vi "AlgorithmLeftGoal - Copy.vi"(0 "MatchBallX":dbl, 1 "MatchBallY":dbl, 2 "D1 X COM":dbl, 3 "D1Y COM":dbl, 4 "D2 X COM":dbl, 5 "D2 Y COM":dbl) -> (9 "RW":cluster{"kRW":dbl, "CoRW":dbl, "type":dbl}, 11 "LW":cluster{"kLW":dbl, "CoLW":dbl, "type":dbl}, 13 "output cluster":T1, 14 "Theta LG,LW":dbl, 15 "aRW":dbl, 16 "aS":dbl, 17 "min x":dbl, 18 "min x2":dbl, 19 "min x3":dbl)   [LabVIEW 2014]
panel:
  out "xD2BotS":dbl
  out "xD2ComS":dbl
  out "xD1BotS":dbl
  out "xD1ComS":dbl
  out "xD2BotR":dbl
  out "xD2ComR":dbl
  out "xD1BotR":dbl
  out "xD1ComR":dbl
  out "D2 X Bot fit 2":dbl
  out "D2 X Com fit":dbl
  out "D1 X Bot fit":dbl
  out "D1 X Com fit":dbl
  # "LOGIC"
  # "Left Goal"
  # "STRAIGHT"
  # "Left wall"
  # "Right Wall"
  # "Straight"
  # "sending data"
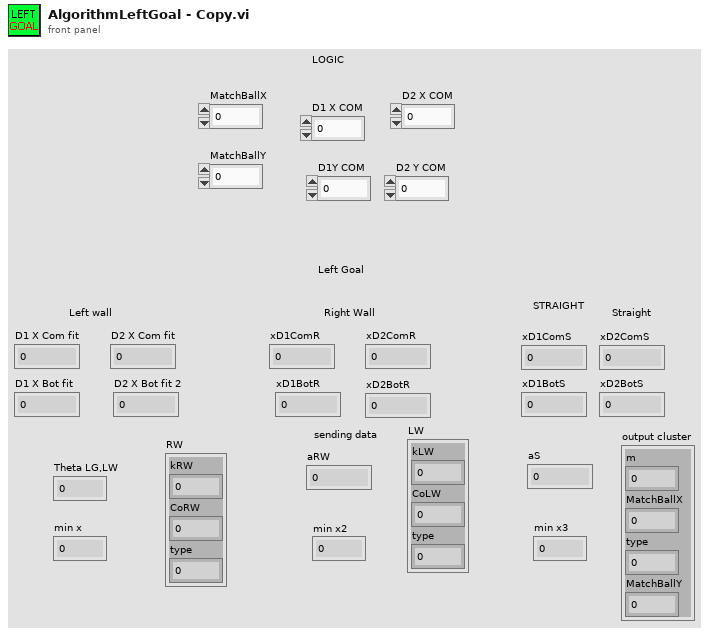
[diagram p1: front panel]
types:
  T1 = cluster{"m":dbl, "MatchBallX":dbl, "type":dbl, "MatchBallY":dbl}
  T2 = cluster{"m":dbl, "MatchBallX":dbl, "y":dbl, "MatchBallY":dbl}
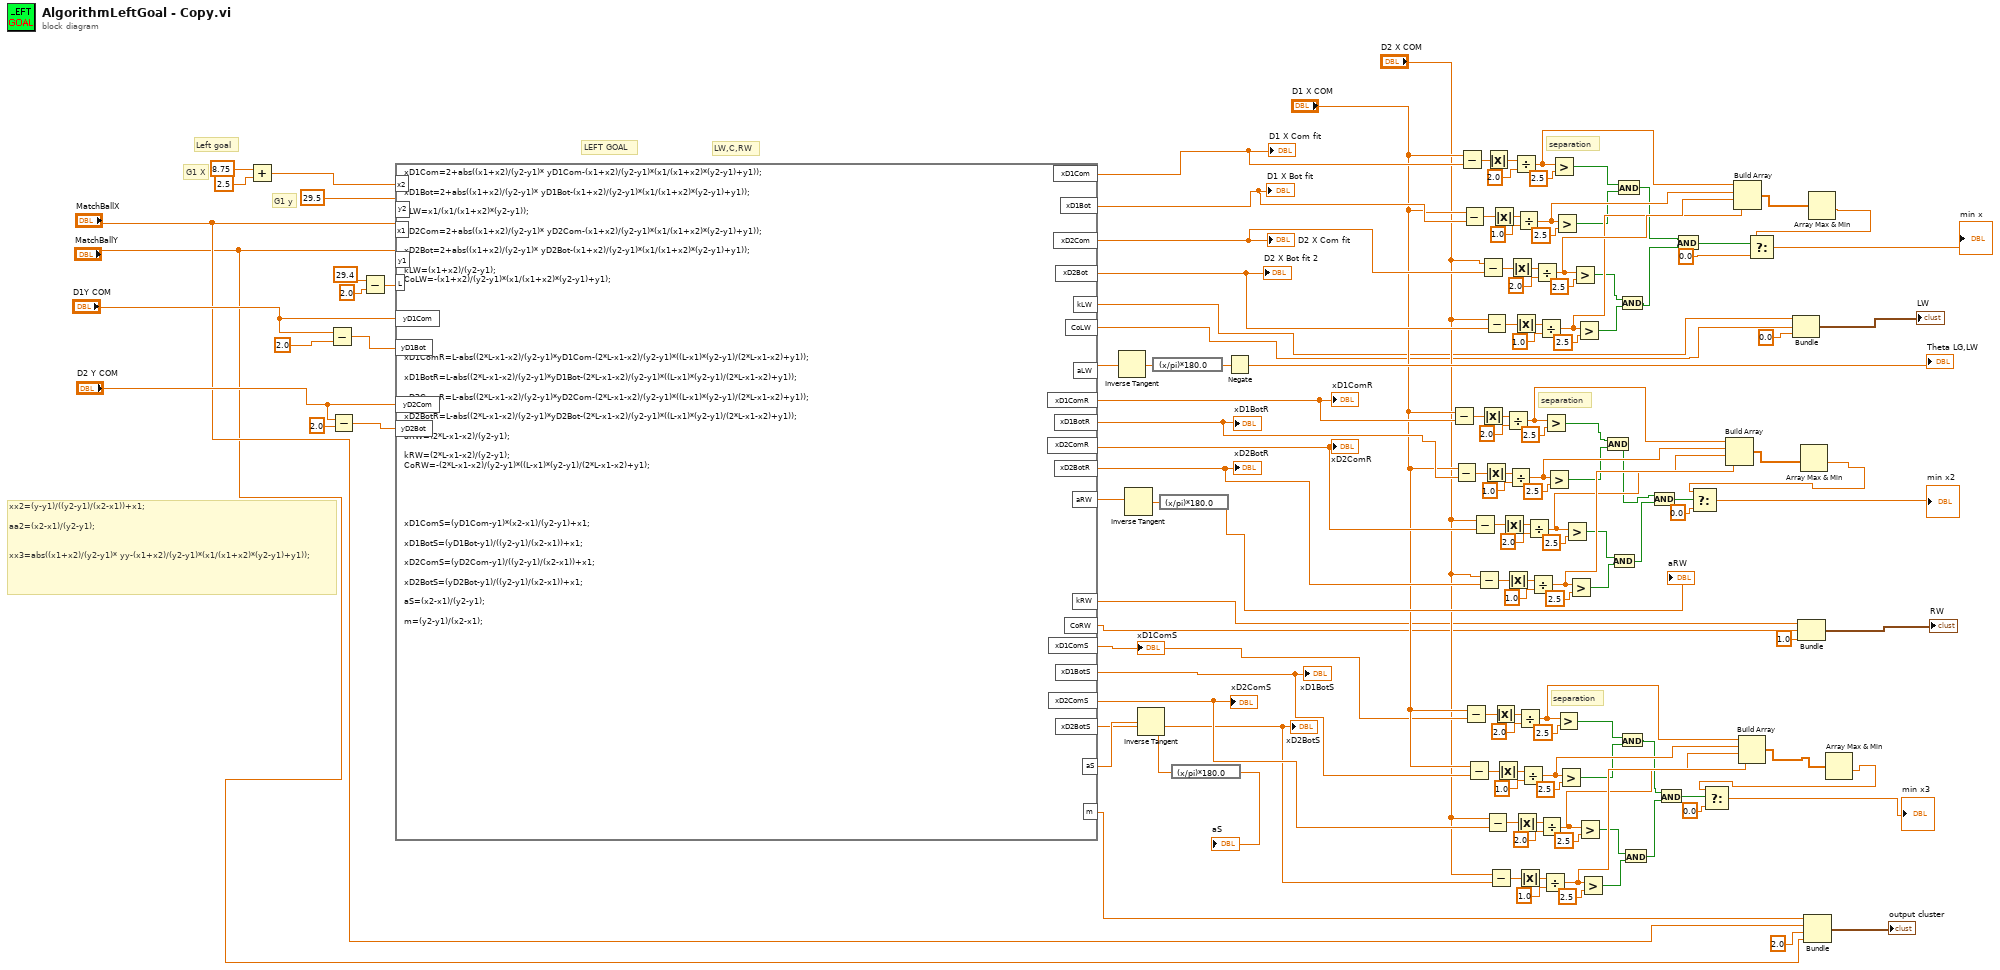
[diagram p0: block diagram]
diagram:
  # "LW,C,RW"
  # "separation"
  # "separation"
  # "separation"
  # "LEFT GOAL"
  # "xx2=(y-y1)/((y2-y1)/(x2-x1))+x1;\n\naa2=(x2-x1)/(y2-y1);\n\n\nxx3=abs((x1+x2)/(y2-y1)* yy-(x1+x2)/(y2-y1)*(x1/(x1+x2)*(y2-y1)+y1));"
  # "Left goal"
  # "G1 y"
  # "G1 X"
  n1 = Add(x=8.75, y=2.5) -> (x+y=w140:dbl)
  n2 = Subtract(x="D1Y COM", y=2.0) -> (x-y=w135:dbl)
  n3 = Subtract(x="D2 Y COM", y=2.0) -> (x-y=w130:dbl)
  n4 = Subtract(x=29.4 ("input variable"), y=2.0) -> (x-y=w15:dbl)
  n5 = formula code="xD1Com=2+abs((x1+x2)/(y2-y1)* yD1Com-(x1+x2)/(y2-y1)*(x1/(x1+x2)*(y2-y1)+y1));\n\nxD1Bot=2+abs((x1+x2)/(y2-y1)* yD1Bot-(x1+x2)/(y2-y1)*(x1/(x1+x2)*(y2-y1)+y1));\n\naLW=x1/(x1/(x1+x2)*(y2-y1));\n\nxD2Com=2+abs((x1+x2)/(y2-y1)* yD2Com-(x1+x2)/(y2-y1)*(x1/(x1+x2)*(y2-y1)+y1));\n\nxD2Bot=2+abs((x1+x2)/(y2-y1)* yD2Bot-(x1+x2)/(y2-y1)*(x1/(x1+x2)*(y2-y1)+y1));\n\nkLW=(x1+x2)/(y2-y1);\nCoLW=-(x1+x2)/(y2-y1)*(x1/(x1+x2)*(y2-y1)+y1);\n\n\n\n\n\n\n\nxD1ComR=L-abs((2*L-x1-x2)/(y2-y1)*yD1Com-(2*L-x1-x2)/(y2-y1)*((L-x1)*(y2-y1)/(2*L-x1-x2)+y1));\n\nxD1BotR=L-abs((2*L-x1-x2)/(y2-y1)*yD1Bot-(2*L-x1-x2)/(y2-y1)*((L-x1)*(y2-y1)/(2*L-x1-x2)+y1));\n\nxD2ComR=L-abs((2*L-x1-x2)/(y2-y1)*yD2Com-(2*L-x1-x2)/(y2-y1)*((L-x1)*(y2-y1)/(2*L-x1-x2)+y1));\n\nxD2BotR=L-abs((2*L-x1-x2)/(y2-y1)*yD2Bot-(2*L-x1-x2)/(y2-y1)*((L-x1)*(y2-y1)/(2*L-x1-x2)+y1));\n\naRW=(2*L-x1-x2)/(y2-y1);\n\nkRW=(2*L-x1-x2)/(y2-y1);\nCoRW=-(2*L-x1-x2)/(y2-y1)*((L-x1)*(y2-y1)/(2*L-x1-x2)+y1);\n\n\n\n\n\nxD1ComS=(yD1Com-y1)*(x2-x1)/(y2-y1)+x1;\n\nxD1BotS=(yD1Bot-y1)/((y2-y1)/(x2-x1))+x1;\n\nxD2ComS=(yD2Com-y1)/((y2-y1)/(x2-x1))+x1;\n\nxD2BotS=(yD2Bot-y1)/((y2-y1)/(x2-x1))+x1;\n\naS=(x2-x1)/(y2-y1);\n\nm=(y2-y1)/(x2-x1);"("x1"="MatchBallX", "x2"=w140, "y2"=29.5, "y1"="MatchBallY", "yD1Com"="D1Y COM", "yD2Com"="D2 Y COM", "yD1Bot"=w135, "yD2Bot"=w130, "L"=w15) -> ("xD1Com"=w123:dbl, "aLW"=w138:dbl, "xD1Bot"=w109:dbl, "xD2Com"=w114:dbl, "xD2Bot"=w104:dbl, "xD1ComR"=w77:dbl, "xD1BotR"=w76:dbl, "xD2ComR"=w75:dbl, "xD2BotR"=w74:dbl, "aRW"=w128:dbl, "xD1ComS"=w51:dbl, "aS"=w124:dbl, "xD1BotS"=w50:dbl, "xD2BotS"=w48:dbl, "xD2ComS"=w49:dbl, "kLW"=w13:dbl, "CoLW"=w12:dbl, "kRW"=w9:dbl, "CoRW"=w8:dbl, "m"=w5:dbl)
  "D1 X Com fit" <- w123
  "D1 X Bot fit" <- w109
  "D2 X Com fit" <- w114
  "D2 X Bot fit 2" <- w104
  "xD1ComR" <- w77
  "xD1BotR" <- w76
  "xD2ComR" <- w75
  "xD2BotR" <- w74
  "xD1ComS" <- w51
  "xD1BotS" <- w50
  "xD2ComS" <- w49
  "xD2BotS" <- w48
  n6 = Inverse Tangent(1:w138) -> (0:w139:dbl)
  n7 = Inverse Tangent(1:w128) -> (0:w129:dbl)
  n8 = Inverse Tangent(1:w124) -> (0:w125:dbl)
  n9 = expression code="(x/pi)*180.0" ("radians to degrees")(w139) -> (w136:dbl)
  n10 = expression code="(x/pi)*180.0" ("radians to degrees")(w129) -> (→"aRW":dbl)
  n11 = expression code="(x/pi)*180.0" ("radians to degrees")(w125) -> (→"aS":dbl)
  n12 = Negate(x=w136) -> (-x=→"Theta LG,LW":dbl)
  n13 = Subtract(x="D1 X COM", y=w77) -> (x-y=w78:dbl)
  n14 = Subtract(x="D1 X COM", y=w76) -> (x-y=w89:dbl)
  n15 = Subtract(x="D1 X COM", y=w123) -> (x-y=w122:dbl)
  n16 = Subtract(x="D1 X COM", y=w109) -> (x-y=w110:dbl)
  n17 = Subtract(x="D1 X COM", y=w51) -> (x-y=w53:dbl)
  n18 = Subtract(x="D1 X COM", y=w50) -> (x-y=w64:dbl)
  n19 = Subtract(x="D2 X COM", y=w75) -> (x-y=w85:dbl)
  n20 = Subtract(x="D2 X COM", y=w74) -> (x-y=w90:dbl)
  n21 = Subtract(x="D2 X COM", y=w114) -> (x-y=w115:dbl)
  n22 = Absolute Value(x=w78) -> (abs(x)=w79:dbl)
  n23 = Absolute Value(x=w89) -> (abs(x)=w88:dbl)
  n24 = Subtract(x="D2 X COM", y=w104) -> (x-y=w108:dbl)
  n25 = Subtract(x="D2 X COM", y=w49) -> (x-y=w60:dbl)
  n26 = Absolute Value(x=w122) -> (abs(x)=w121:dbl)
  n27 = Subtract(x="D2 X COM", y=w48) -> (x-y=w65:dbl)
  n28 = Absolute Value(x=w110) -> (abs(x)=w111:dbl)
  n29 = Absolute Value(x=w53) -> (abs(x)=w54:dbl)
  n30 = Absolute Value(x=w64) -> (abs(x)=w63:dbl)
  n31 = Absolute Value(x=w85) -> (abs(x)=w84:dbl)
  n32 = Divide(x=w79, y=2.0) -> (x/y=w95:dbl)
  n33 = Absolute Value(x=w90) -> (abs(x)=w91:dbl)
  n34 = Divide(x=w88, y=1.0) -> (x/y=w96:dbl)
  n35 = Absolute Value(x=w115) -> (abs(x)=w116:dbl)
  n36 = Divide(x=w121, y=2.0) -> (x/y=w102:dbl)
  n37 = Absolute Value(x=w108) -> (abs(x)=w107:dbl)
  n38 = Absolute Value(x=w60) -> (abs(x)=w59:dbl)
  n39 = Divide(x=w111, y=1.0) -> (x/y=w101:dbl)
  n40 = Divide(x=w54, y=2.0) -> (x/y=w70:dbl)
  n41 = Absolute Value(x=w65) -> (abs(x)=w66:dbl)
  n42 = Divide(x=w63, y=1.0) -> (x/y=w71:dbl)
  n43 = Divide(x=w84, y=2.0) -> (x/y=w97:dbl)
  n44 = Divide(x=w91, y=1.0) -> (x/y=w98:dbl)
  n45 = Divide(x=w116, y=2.0) -> (x/y=w100:dbl)
  n46 = Divide(x=w107, y=1.0) -> (x/y=w99:dbl)
  n47 = Divide(x=w59, y=2.0) -> (x/y=w72:dbl)
  n48 = Divide(x=w66, y=1.0) -> (x/y=w73:dbl)
  n49 = Greater?(x=w95, y=2.5) -> (0:w34:bool)
  n50 = Greater?(x=w96, y=2.5) -> (0:w33:bool)
  n51 = Greater?(x=w102, y=2.5) -> (0:w39:bool)
  n52 = Greater?(x=w101, y=2.5) -> (0:w38:bool)
  n53 = Greater?(x=w70, y=2.5) -> (0:w29:bool)
  n54 = Greater?(x=w71, y=2.5) -> (0:w28:bool)
  n55 = Greater?(x=w97, y=2.5) -> (0:w32:bool)
  n56 = Greater?(x=w98, y=2.5) -> (0:w31:bool)
  n57 = Greater?(x=w100, y=2.5) -> (0:w43:bool)
  n58 = Greater?(x=w99, y=2.5) -> (0:w42:bool)
  n59 = Greater?(x=w72, y=2.5) -> (0:w26:bool)
  n60 = Greater?(x=w73, y=2.5) -> (0:w25:bool)
  n61 = And(x=w34, y=w33) -> (x .and. y?=w35:bool)
  n62 = And(x=w32, y=w31) -> (x .and. y?=w30:bool)
  n63 = And(x=w39, y=w38) -> (x .and. y?=w37:bool)
  n64 = And(x=w43, y=w42) -> (x .and. y?=w40:bool)
  n65 = And(x=w29, y=w28) -> (x .and. y?=w27:bool)
  n66 = And(x=w26, y=w25) -> (x .and. y?=w24:bool)
  n67 = And(x=w35, y=w30) -> (x .and. y?=w36:bool)
  n68 = And(x=w27, y=w24) -> (x .and. y?=w23:bool)
  n69 = And(x=w37, y=w40) -> (x .and. y?=w41:bool)
  n70 = Build Array(w95, w96, w97, w98) -> (w20:dbl[])
  n71 = Build Array(w102, w101, w100, w99) -> (w22:dbl[])
  n72 = Build Array(w70, w71, w72, w73) -> (w18:dbl[])
  n73 = Bundle("kLW"=w13, "CoLW"=w12, "y"=0.0) -> (→"LW":cluster{"kLW":dbl, "CoLW":dbl, "y":dbl})  [unwired: 1 in]
  n74 = Bundle("kRW"=w9, "CoRW"=w8, "y"=1.0) -> (→"RW":cluster{"kRW":dbl, "CoRW":dbl, "y":dbl})  [unwired: 1 in]
  n75 = Array Max & Min(array=w20) -> (min value=w19:dbl)  [unwired: 3 out]
  n76 = Select(t=w19, s=w36, f=0.0 ("y")) -> (s? t:f=→"min x2":dbl)
  n77 = Bundle("m"=w5, "MatchBallX"="MatchBallX", "y"=2.0, "MatchBallY"="MatchBallY") -> (→"output cluster":T2)  [unwired: 1 in]
  n78 = Array Max & Min(array=w22) -> (min value=w21:dbl)  [unwired: 3 out]
  n79 = Select(t=w21, s=w41, f=0.0 ("y")) -> (s? t:f=→"min x":dbl)
  n80 = Array Max & Min(array=w18) -> (min value=w17:dbl)  [unwired: 3 out]
  n81 = Select(t=w17, s=w23, f=0.0 ("y")) -> (s? t:f=→"min x3":dbl)
